vi "FM Radio.vi"() -> ()   [LabVIEW 2021]
uses:
  <vilib>/Analysis/3filter.llb/Filter Passband Type.ctl
  <vilib>/Analysis/2dsp.llb/Complex FFT.vi
  <vilib>/Analysis/2dsp.llb/Inverse Complex FFT.vi
  <vilib>/Analysis/2dsp.llb/Decimate (single shot, CDB).vi
  <vilib>/Analysis/2dsp.llb/1D Convolution (DBL).vi
  <vilib>/Analysis/2dsp.llb/Decimate (single shot, DBL).vi
  VIs/Initialize by Serial.vi
  VIs/Read DBL.vi
  RTL-SDR.lvlib
  <vilib>/Analysis/NI_AALPro.lvlib
  <vilib>/Analysis/NI_AALBase.lvlib
  <vilib>/ptbypt/NI_PtbyPt.lvlib
panel:
  out "Output Graph":waveform(dbl)(graph)
  in  "output path":path=path "/home/jhpaques/Git/jhpaques/RTL_SDR/output.wav"
  out "XY Graph":cluster{"X":dbl, "Y":dbl}[](graph)
  out "# samples":i32
  in  "record time (s)":dbl=1.0 format="%#_13g"
  out "Waveform Graph":waveform(dbl)[](graph)=[{"t0"=timestamp(0 s since 1904-01-01), "dt"=5e-07, "Y"=[]}, {"t0"=timestamp(0 s since 1904-01-01), "dt"=5e-07, "Y"=[]}]
  out "FFT Graph":cluster{"f0":dbl, "df":dbl, "Y":dbl[]}(graph)={"f0"=nan, "df"=inf, "Y"=[]}
  out "error out":errorcluster
  in  "FFT size":i32=8192
  out "Actual Sample Rate (Hz)":u32 format="%#.6p"
  in  "Sample Rate (Hz)":u32=2400000 format="%#.6p"
  out "Manufacturer Name":string="Realtek"
  out "Product Name":string="RTL2838UHIDIR"
  out "Serial Number":string="00000001"
  in  "Center Frequency (Hz)":u32=87800000 format="%#_6p"
  out "Actual Center Frequency (Hz)":u32 format="%#.6p"
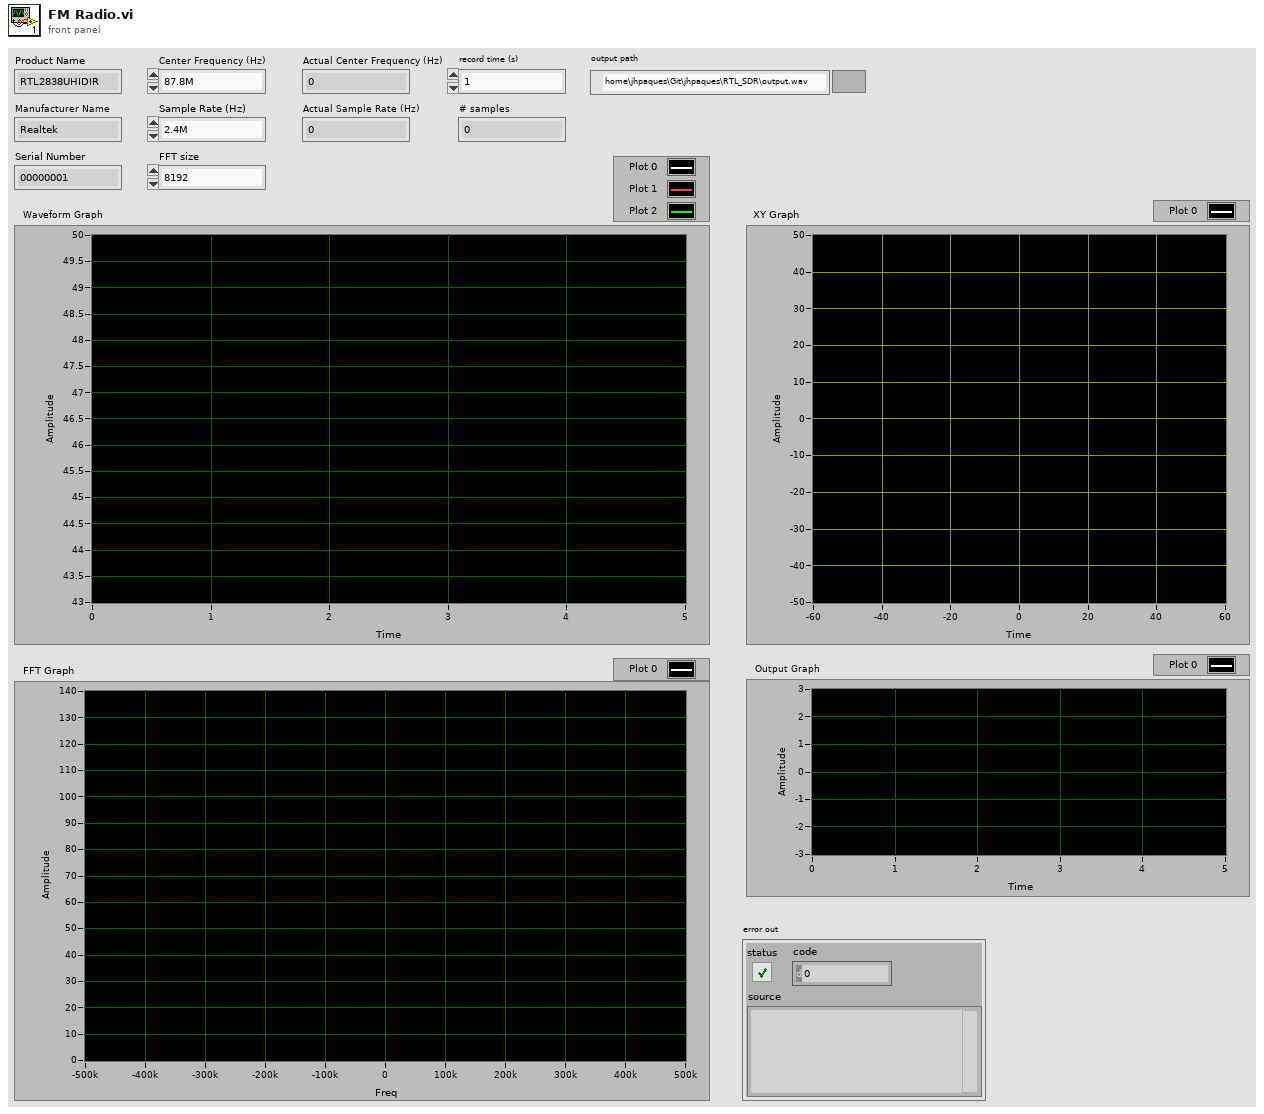
[diagram p1: front panel]
types:
  T1 = typedef "RTL-SDR.lvlib/Device Handle.ctl" = u64
  T2 = typedef "NI_AALBase.lvlib/Filter Passband Type.ctl" = enum32{"Lowpass", "Highpass", "Bandpass", "Bandstop"}
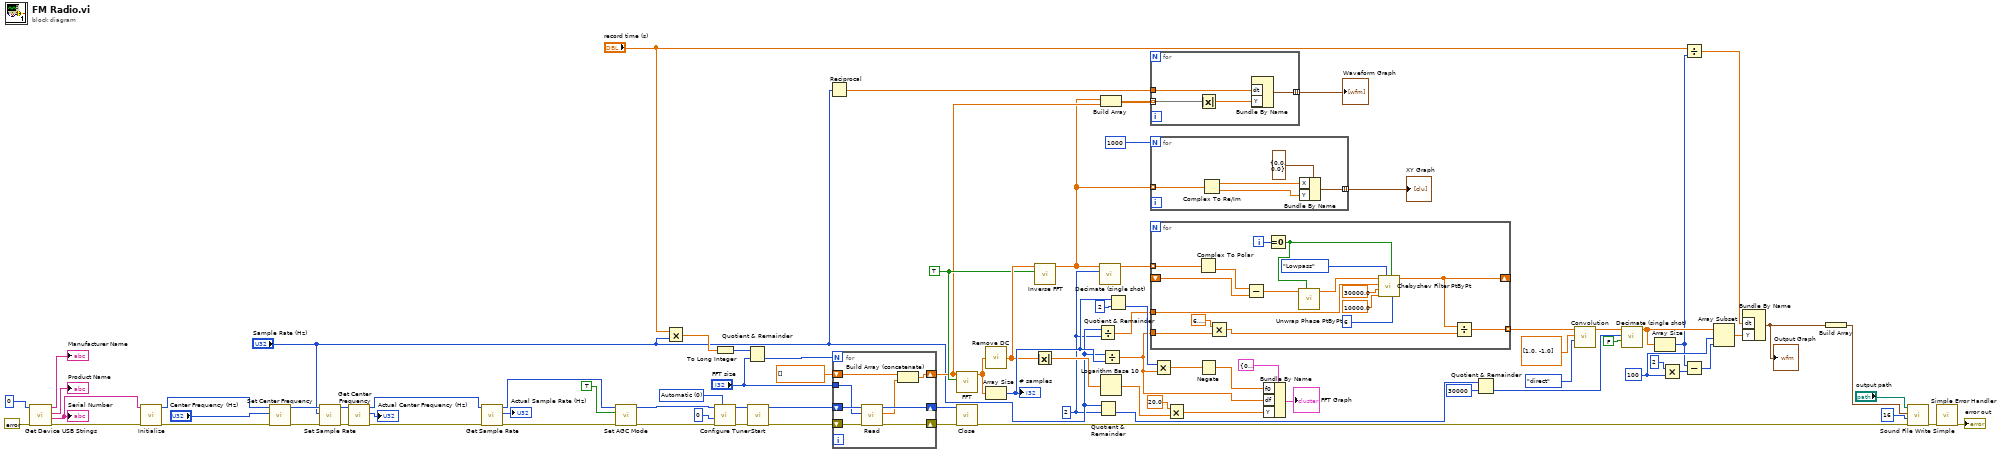
[diagram p0: block diagram]
diagram:
  w7 = 2 ("decimating factor")
  w9 = 100 ("y")
  w38 = TRUE ("shift?")
  w67 = u16 0 items=["Automatic", "Manual"] ("Tuner Gain Mode")
  n1 = call "Get Device USB Strings.vi"("error in (no error)"=errorcluster {"status"=FALSE, "code"=0, "source"=""} ("error in"), "device index"=u32 0) -> ("error out"=w84:errorcluster, "Serial Number"=w80:string, "Product Name"=→"Product Name":string, "Manufacturer Name"=→"Manufacturer Name":string)  [unwired: 6 in]
  "Serial Number" <- w80
  n2 = call-poly "Initialize.vi"("error in (no error)"=w84, "Serial Number"=w80) -> ("error out"=w77:errorcluster, "device handle out"=w78:T1)  [unwired: 8 in]
  n3 = call "Set Center Frequency.vi"("error in (no error)"=w77, "Center Frequency (Hz)"="Center Frequency (Hz)", "device handle in"=w78) -> ("error out"=w58:errorcluster, "device handle out"=w59:T1)  [unwired: 7 in]
  n4 = call "Set Sample Rate.vi"("error in (no error)"=w58, "Sample Rate (Hz)"="Sample Rate (Hz)", "device handle in"=w59) -> ("error out"=w74:errorcluster, "device handle out"=w73:T1)  [unwired: 7 in]
  n5 = call "Get Center Frequency.vi"("error in (no error)"=w74, "device handle in"=w73) -> ("error out"=w60:errorcluster, "Center Frequency (Hz)"=→"Actual Center Frequency (Hz)":u32, "device handle out"=w61:T1)  [unwired: 7 in]
  n6 = call "Get Sample Rate.vi"("error in (no error)"=w60, "device handle in"=w61) -> ("error out"=w64:errorcluster, "Sample Rate (Hz)"=→"Actual Sample Rate (Hz)":u32, "device handle out"=w65:T1)  [unwired: 7 in]
  n7 = call "Set AGC Mode.vi"("error in (no error)"=w64, "Enable AGC (T)"=TRUE, "device handle in"=w65) -> ("error out"=w70:errorcluster, "device handle out"=w69:T1)  [unwired: 7 in]
  n8 = Multiply(x="record time (s)", y="Sample Rate (Hz)") -> (x*y=w35:dbl)
  n9 = To Long Integer(number=w35) -> (32bit integer=w32:i32)
  n10 = call "Configure Tuner.vi"("Tuner Gain Mode (0: auto)"=w67, "error in (no error)"=w70, "Bandwidth (Hz) (0: auto)"=u32 0, "device handle in"=w69) -> ("error out"=w63:errorcluster, "device handle out"=w56:T1)  [unwired: 6 in]
  n11 = Quotient & Remainder(x=w32, y="FFT size") -> (floor(x/y)=w34:i32)  [unwired: 1 out]
  n12 = call "Start.vi"("error in (no error)"=w63, "device handle in"=w56) -> ("error out"=w75:errorcluster, "device handle out"=w55:T1)  [unwired: 8 in]
  n13 = Reciprocal(x="Sample Rate (Hz)") -> (1/x=w41:dbl)
  n14 = for {
    N: w34 -> [_]
    tunnel: "FFT size" -> [w89]
    shift-right: [w93] -> w79
    shift-left: w75 -> [w92]
    shift-right: [w91] -> w57
    shift-left: w55 -> [w90]
    shift-right: [w86] -> w36
    shift-left: cdb[] [] -> [w87]
    n15 = call-poly "Read.vi"("error in (no error)"=w92, "# samples"=w89, "device handle in"=w90) -> ("error out"=w93:errorcluster, "Data"=w88:cdb[], "device handle out"=w91:T1)  [unwired: 6 in]
    n16 = Build Array (concatenate)(w87, w88) -> (w86:cdb[])
  }
  n17 = call-poly <vilib>:"FFT.vi"("shift?"=w38, "X"=w36) -> ("FFT {X}"=w46:cdb[])  [unwired: 8 in, 1 out]
  n18 = call "Close.vi"("error in"=w79, "device handle in"=w57) -> ("error out"=w29:errorcluster)  [unwired: 9 in]
  n19 = call "Remove DC.vi"("FFT in"=w46) -> ("FFT out"=w39:cdb[])
  n20 = Array Size(array=w46) -> (size(s)=w48:i32)
  "# samples" <- w48
  n21 = Absolute Value(x=w39) -> (abs(x)=w43:dbl[])
  n22 = call-poly <vilib>:"Inverse FFT.vi"("shift?"=w38, "FFT {X}"=w39) -> ("X"=w17:cdb[])  [unwired: 8 in, 1 out]
  n23 = Divide(x="Sample Rate (Hz)", y=w7) -> (x/y=w6:dbl)
  n24 = Quotient & Remainder(x="Sample Rate (Hz)", y=w7) -> (floor(x/y)=w15:u32)  [unwired: 1 out]
  n25 = call-poly <vilib>:"Decimate (single shot).vi"("decimating factor"=w7, "X"=w17) -> ("Decimated Array"=w16:cdb[])  [unwired: 8 in, 1 out]
  n26 = Build Array(w17, w36) -> (w37:cdb[][])
  n27 = Logarithm Base 10(1:w43) -> (0:w45:dbl[])
  n28 = Divide(x="Sample Rate (Hz)", y=w48) -> (x/y=w21:dbl)
  n29 = Quotient & Remainder(x=w48, y=2) -> (floor(x/y)=w49:i32)  [unwired: 1 out]
  n30 = for {
    tunnel: w41 -> [w97]
    tunnel: [w96] -> w40 mode=indexing
    tunnel: w37 -> [w94] mode=indexing
    n31 = Absolute Value(x=w94) -> (abs(x)=w95:dbl[])
    n32 = Bundle By Name("dt"=w97, "Y"=w95) -> (w96:waveform(dbl))  [unwired: 1 in]
  }
  "Waveform Graph" <- w40
  n33 = for {
    N: 1000 -> [_]
    tunnel: [w102] -> w31 mode=indexing
    tunnel: w17 -> [w98] mode=indexing
    n34 = Complex To Re/Im(x + iy=w98) -> (x=w100:dbl, y=w99:dbl)
    n35 = Bundle By Name(cluster=cluster{"X":dbl, "Y":dbl} {"X"=0.0, "Y"=0.0} ("XY Graph"), "X"=w100, "Y"=w99) -> (w102:cluster{"X":dbl, "Y":dbl})
  }
  "XY Graph" <- w31
  n36 = for {
    shift-right: [w110] -> _
    shift-left: _ -> [w118]
    tunnel: w16 -> [w117] mode=indexing
    tunnel: w6 -> [w116]
    tunnel: [w109] -> w5 mode=indexing
    tunnel: w21 -> [w106]
    i -> [w111]
    n37 = Complex To Polar(r * e^(i*theta)=w117) -> (theta=w119:dbl)  [unwired: 1 out]
    n38 = Multiply(x=6.283185307179586, y=w106) -> (x*y=w108:dbl)
    n39 = Subtract(x=w119, y=w118) -> (x-y=w104:dbl)
    n40 = Equal To 0?(x=w111) -> (x = 0?=w103:bool)
    n41 = call <vilib>:"Unwrap Phase PtByPt.vi"("initialize"=w103, "phase"=w104) -> ("unwrapped phase"=w105:dbl)  [unwired: 9 in]
    n42 = call <vilib>:"Chebyshev Filter PtByPt.vi"("order"=6, "initialize"=w103, "filter type"=Filter_Passband_Type."Lowpass", "low cutoff freq: fl"=10000.0, "high cutoff freq: fh"=30000.0, "sampling freq: fs"=w116, "x"=w105) -> ("Filtered x"=w110:dbl)  [unwired: 3 in, 1 out]
    n43 = Divide(x=w110, y=w108) -> (x/y=w109:dbl)
  }
  n44 = Multiply(x=w49, y=w21) -> (x*y=w50:dbl)
  n45 = Multiply(x=20.0, y=w45) -> (x*y=w42:dbl[])
  n46 = Negate(x=w50) -> (-x=w47:dbl)
  n47 = Bundle By Name(cluster=cluster{"f0":dbl, "df":dbl, "Y":dbl[]} {"f0"=0.0, "df"=0.0, "Y"=[]}, "f0"=w47, "df"=w21, "Y"=w42) -> (→"FFT Graph":cluster{"f0":dbl, "df":dbl, "Y":dbl[]})
  n48 = Quotient & Remainder(x=w15, y=30000) -> (floor(x/y)=w25:u32)  [unwired: 1 out]
  n49 = call-poly <vilib>:"Convolution.vi"("algorithm"=enum32{"direct", "frequency domain"}."direct", "Y"=dbl[] [1.0, -1.0], "X"=w5) -> ("X * Y"=w4:dbl[])  [unwired: 7 in, 1 out]
  n50 = call-poly <vilib>:"Decimate (single shot).vi"("averaging"=FALSE, "decimating factor"=w25, "X"=w4) -> ("Decimated Array"=w14:dbl[])  [unwired: 7 in, 1 out]
  n51 = Array Size(array=w14) -> (size(s)=w2:i32)
  n52 = Multiply(x=2, y=w9) -> (x*y=w11:i32)
  n53 = Divide(x="record time (s)", y=w2) -> (x/y=w3:dbl)
  n54 = Subtract(x=w2, y=w11) -> (x-y=w18:i32)
  n55 = Array Subset(array=w14, index=w9, length=w18) -> (w13:dbl[])
  n56 = Bundle By Name("dt"=w3, "Y"=w13) -> (w20:waveform(dbl))  [unwired: 1 in]
  "Output Graph" <- w20
  n57 = Build Array(w20) -> (w23:waveform(dbl)[])
  n58 = call <vilib>:"Sound File Write Simple.vi"("error in (no error)"=w29, "bits per sample"=16, "data"=w23, "path"="output path") -> ("error out"=w28:errorcluster)  [unwired: 6 in, 1 out]
  n59 = call <vilib>:"Simple Error Handler.vi"("error in (no error)"=w28) -> ("error out"=→"error out":errorcluster)  [unwired: 4 in, 4 out]
